vi "Untitled 1.vi"() -> ()   [LabVIEW 2014]
panel:
  out "Array 2":u32[][](array[numeric]) format="%x"
  out "Array":dbl[](array[numeric])
  out "Image Pixels (U32) 2":u32[][](array[colorbox])
  out "Image Pixels (U32)":u32[][](array[colorbox])
  in  "Stop (F)":bool
  out "Image Out":T1(plugin-control)
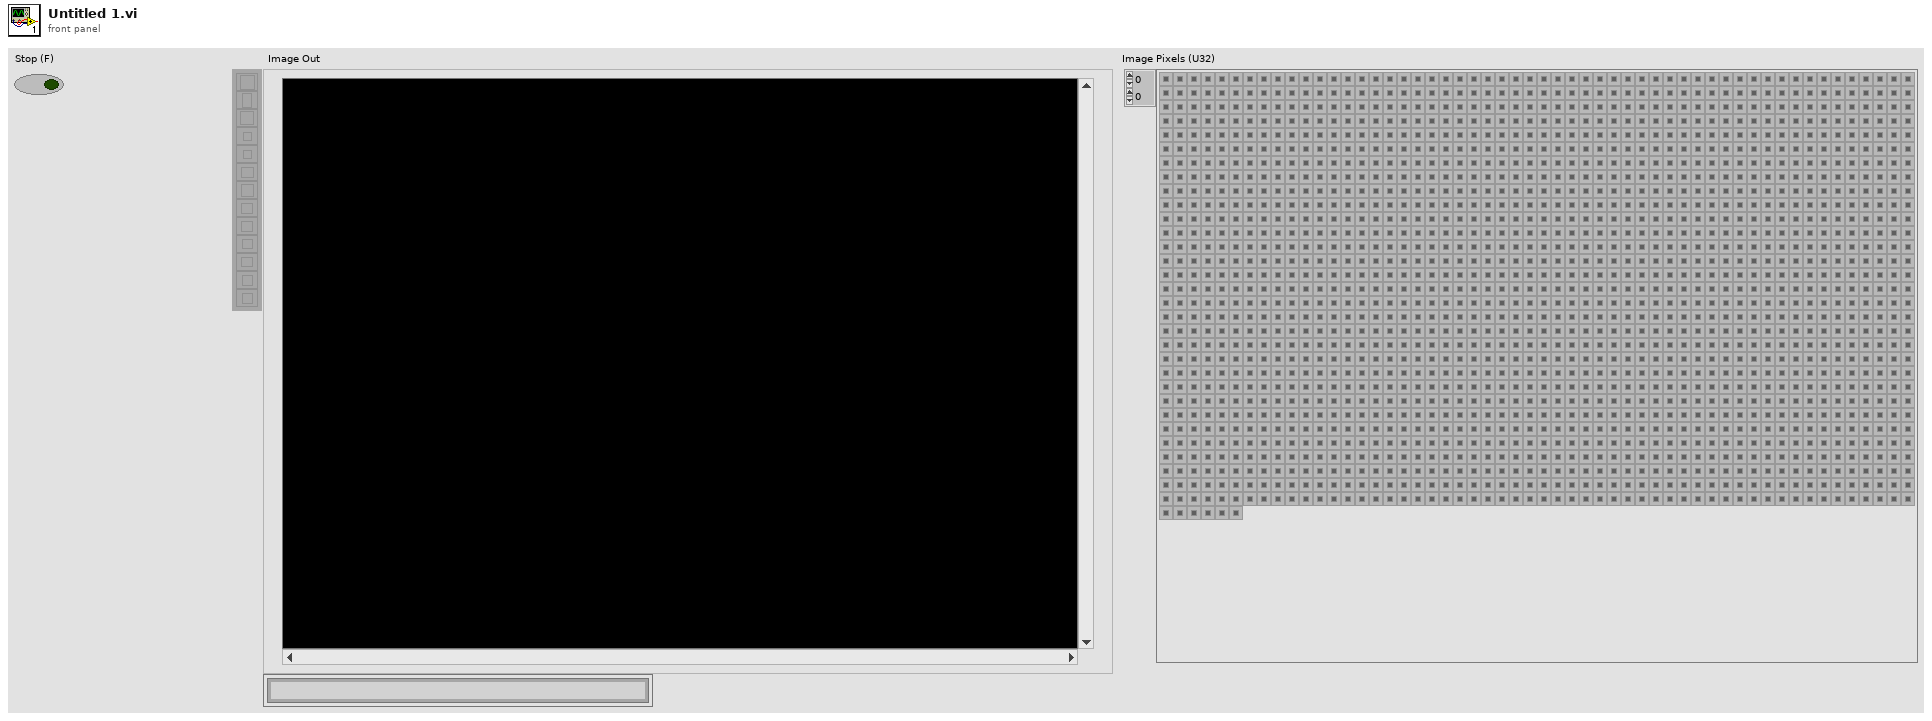
[diagram p1: front panel]
types:
  T1 = typedef "IMAQ Image.ctl" = refnum<image>
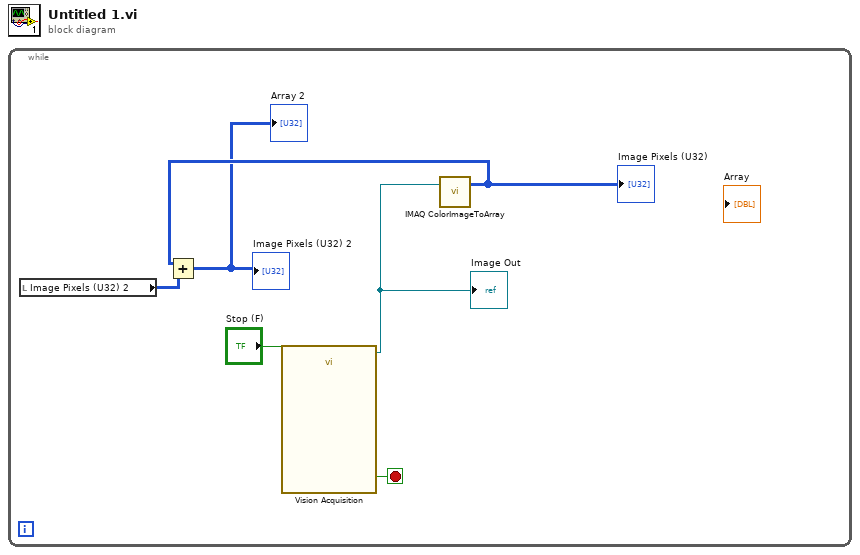
[diagram p0: block diagram]
diagram:
  n1 = while {
    stop <- w5 stop-if-true
    n2 = local read "Image Pixels (U32) 2"() -> (w3:u32[][])
    n3 = call "Vision Acquisition"("Stop (F)"="Stop (F)") -> ("Image Out"=w4:T1, "Stopped"=w5:bool)  [unwired: 24 in, 1 out]
    "Image Out" <- w4
    n4 = call "IMAQ ColorImageToArray"("Image"=w4) -> ("Image Pixels (U32)"=w2:u32[][])  [unwired: 3 in, 2 out]
    "Image Pixels (U32)" <- w2
    n5 = Add(x=w2, y=w3) -> (x+y=→"Image Pixels (U32) 2" →"Array 2":u32[][])
  }
